vi "UI_Set_Stop_State_(04A).vi"(3 "error in (no error)":errorcluster, 4 "Settings cluster in":T1={"Defaults"={"Default User"=0.0, "VISA Resource Name "=""}, "Recording and saving"={"Researcher name"="", "Name prefix"="", "Data filtering"=0, "Stop at"=0.0, "\"Stop at\" enabled"=FALSE}, "Geometry"={"Cage diameter, mm"=0, "Starting angle MIDFIELD"=0, "Starting angle BORDER"=0, "Radius, mm CENTER"=0, "Radius, mm MIDFIELD"=0, "N segments MIDFIELD"=0, "N segments BORDER"=0, "R-gap, mm"=0.0, "Bridge swap"=FALSE, "Bridge H. offset"=0.0, "Bridge V. offset"=0.0, "Twisted neck"=FALSE, "Alt. magn. orientation"=FALSE}, "IO parameters"={"IO general config."=0, "IO 1 configuration"=0, "IO 2 configuration"=0, "IO 3 configuration"=0, "IO 4 configuration"=0, "Activate ext. RS-232"=0, "IO inversion config."=0, "Sync capability"=1}, "Stimulus presets array"=[{"Event type"=0, "Dur., s"=0.0, "Stim., s"=0.0, "TTL out N"=1, "Set/Clear"=FALSE, "Stim. has been set"=FALSE}, {"Event type"=0, "Dur., s"=0.0, "Stim., s"=0.0, "TTL out N"=1, "Set/Clear"=FALSE, "Stim. has been set"=FALSE}, {"Event type"=0, "Dur., s"=0.0, "Stim., s"=0.0, "TTL out N"=1, "Set/Clear"=FALSE, "Stim. has been set"=FALSE}, {"Event type"=0, "Dur., s"=0.0, "Stim., s"=0.0, "TTL out N"=1, "Set/Clear"=FALSE, "Stim. has been set"=FALSE}, {"Event type"=0, "Dur., s"=0.0, "Stim., s"=0.0, "TTL out N"=1, "Set/Clear"=FALSE, "Stim. has been set"=FALSE}, {"Event type"=0, "Dur., s"=0.0, "Stim., s"=0.0, "TTL out N"=1, "Set/Clear"=FALSE, "Stim. has been set"=FALSE}, {"Event type"=0, "Dur., s"=0.0, "Stim., s"=0.0, "TTL out N"=1, "Set/Clear"=FALSE, "Stim. has been set"=FALSE}, {"Event type"=0, "Dur., s"=0.0, "Stim., s"=0.0, "TTL out N"=1, "Set/Clear"=FALSE, "Stim. has been set"=FALSE}, {"Event type"=0, "Dur., s"=0.0, "Stim., s"=0.0, "TTL out N"=1, "Set/Clear"=FALSE, "Stim. has been set"=FALSE}, {"Event type"=0, "Dur., s"=0.0, "Stim., s"=0.0, "TTL out N"=1, "Set/Clear"=FALSE, "Stim. has been set"=FALSE}, {"Event type"=0, "Dur., s"=0.0, "Stim., s"=0.0, "TTL out N"=1, "Set/Clear"=FALSE, "Stim. has been set"=FALSE}, {"Event type"=0, "Dur., s"=0.0, "Stim., s"=0.0, "TTL out N"=1, "Set/Clear"=FALSE, "Stim. has been set"=FALSE}, {"Event type"=0, "Dur., s"=0.0, "Stim., s"=0.0, "TTL out N"=1, "Set/Clear"=FALSE, "Stim. has been set"=FALSE}, {"Event type"=0, "Dur., s"=0.0, "Stim., s"=0.0, "TTL out N"=1, "Set/Clear"=FALSE, "Stim. has been set"=FALSE}], "Settings loaded OK"=FALSE} {"Stimulus presets array"."Event type" items=["Stay for N seconds"]; "Stimulus presets array"."TTL out N" items=["1"=1, "2"=2, "1+2"=3]; "Geometry"."Cage diameter, mm" scale=0.0..340.0}, 5 "All references in":T7) -> (0 "error out":errorcluster, 1 "Settings cluster out":T1={"Defaults"={"Default User"=0.0, "VISA Resource Name "=""}, "Recording and saving"={"Researcher name"="", "Name prefix"="", "Data filtering"=0, "Stop at"=0.0, "\"Stop at\" enabled"=FALSE}, "Geometry"={"Cage diameter, mm"=0, "Starting angle MIDFIELD"=0, "Starting angle BORDER"=0, "Radius, mm CENTER"=0, "Radius, mm MIDFIELD"=0, "N segments MIDFIELD"=0, "N segments BORDER"=0, "R-gap, mm"=0.0, "Bridge swap"=FALSE, "Bridge H. offset"=0.0, "Bridge V. offset"=0.0, "Twisted neck"=FALSE, "Alt. magn. orientation"=FALSE}, "IO parameters"={"IO general config."=0, "IO 1 configuration"=0, "IO 2 configuration"=0, "IO 3 configuration"=0, "IO 4 configuration"=0, "Activate ext. RS-232"=0, "IO inversion config."=0, "Sync capability"=1}, "Stimulus presets array"=[{"Event type"=0, "Dur., s"=0.0, "Stim., s"=0.0, "TTL out N"=1, "Set/Clear"=FALSE, "Stim. has been set"=FALSE}, {"Event type"=0, "Dur., s"=0.0, "Stim., s"=0.0, "TTL out N"=1, "Set/Clear"=FALSE, "Stim. has been set"=FALSE}, {"Event type"=0, "Dur., s"=0.0, "Stim., s"=0.0, "TTL out N"=1, "Set/Clear"=FALSE, "Stim. has been set"=FALSE}, {"Event type"=0, "Dur., s"=0.0, "Stim., s"=0.0, "TTL out N"=1, "Set/Clear"=FALSE, "Stim. has been set"=FALSE}, {"Event type"=0, "Dur., s"=0.0, "Stim., s"=0.0, "TTL out N"=1, "Set/Clear"=FALSE, "Stim. has been set"=FALSE}, {"Event type"=0, "Dur., s"=0.0, "Stim., s"=0.0, "TTL out N"=1, "Set/Clear"=FALSE, "Stim. has been set"=FALSE}, {"Event type"=0, "Dur., s"=0.0, "Stim., s"=0.0, "TTL out N"=1, "Set/Clear"=FALSE, "Stim. has been set"=FALSE}, {"Event type"=0, "Dur., s"=0.0, "Stim., s"=0.0, "TTL out N"=1, "Set/Clear"=FALSE, "Stim. has been set"=FALSE}, {"Event type"=0, "Dur., s"=0.0, "Stim., s"=0.0, "TTL out N"=1, "Set/Clear"=FALSE, "Stim. has been set"=FALSE}, {"Event type"=0, "Dur., s"=0.0, "Stim., s"=0.0, "TTL out N"=1, "Set/Clear"=FALSE, "Stim. has been set"=FALSE}, {"Event type"=0, "Dur., s"=0.0, "Stim., s"=0.0, "TTL out N"=1, "Set/Clear"=FALSE, "Stim. has been set"=FALSE}, {"Event type"=0, "Dur., s"=0.0, "Stim., s"=0.0, "TTL out N"=1, "Set/Clear"=FALSE, "Stim. has been set"=FALSE}, {"Event type"=0, "Dur., s"=0.0, "Stim., s"=0.0, "TTL out N"=1, "Set/Clear"=FALSE, "Stim. has been set"=FALSE}, {"Event type"=0, "Dur., s"=0.0, "Stim., s"=0.0, "TTL out N"=1, "Set/Clear"=FALSE, "Stim. has been set"=FALSE}], "Settings loaded OK"=FALSE} {"Stimulus presets array"."Event type" items=["Stay for N seconds"]; "Stimulus presets array"."TTL out N" items=["1"=1, "2"=2, "1+2"=3]; "Geometry"."Cage diameter, mm" scale=0.0..340.0}, 2 "All references out":T7)   [LabVIEW 2018]
uses:
  Controls/CTL_All_References.ctl
  Controls/CTL_Controls_References.ctl
  Controls/CTL_Indicators_References.ctl
  Controls/CTL_Panes_and_VIs_References.ctl
  Controls/CTL_Histogram_Properties.ctl
  <vilib>/Utility/miscctls.llb/LVRangeTypeDef.ctl
  Controls/CTL_Settings_cluster.ctl
  Controls/CTL_Segmented_plot_parameters.ctl
  Controls/CTL_IO_params_cluster.ctl
  Controls/CTL_Single_stimulus_setting.ctl
  <vilib>/Utility/error.llb/Error Cluster From Error Code.vi
  <vilib>/ErrorRing/Error Ring.xnode
panel:
  in  "Histogram initialization cluster":T5={"X Scale.Range"={"Minimum"=0.0, "Maximum"=13.0, "Increment"=1.0, "Minor Increment"=1.0, "Start"=0.0}, "Caption.Text"="Zone preference (normalized)", "X Scale.Offset and Multiplier:Multiplier"=1.0, "X Scale.Offset and Multiplier:Offset"=0.0, "X Scale.Scale Fit"=2, "X Scale.Display Format:Precision"=0, "Y Scale.Mapping Mode"=0, "Zones preference empty initialized array"=[0, 0, 0, 0, 0, 0, 0, 0, 0, 0, 0, 0, 0, 0], "Plot.Fill/Point Color"=15790320}
  out "Panes references":T10
  out "Controls references params":string[][](array[string])
  out "Indicators references params":string[][](array[string])
  out "Indicators references":T9
  out "Controls references":T8
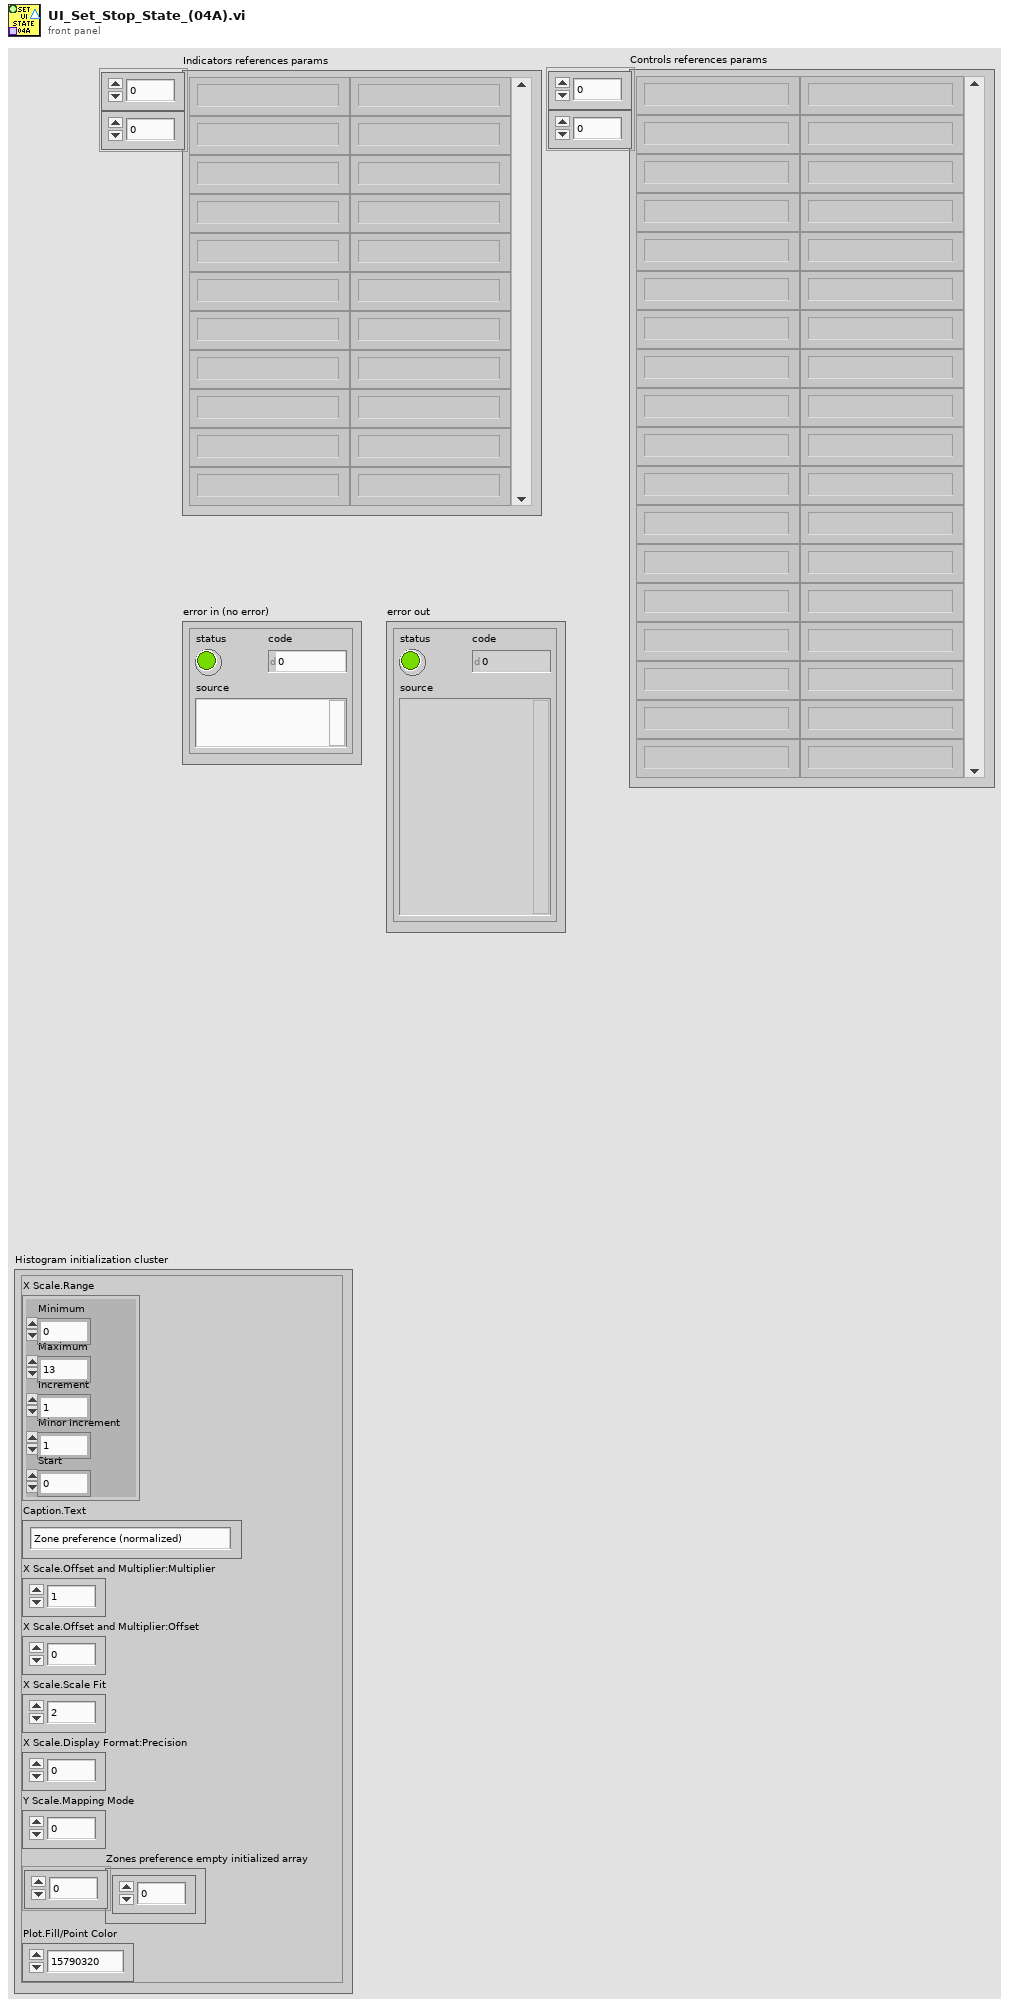
[diagram p1: front panel]
types:
  T1 = typedef "CTL_Settings_cluster.ctl" = cluster{"Defaults":cluster{"Default User":dbl, "VISA Resource Name ":string}, "Recording and saving":cluster{"Researcher name":string, "Name prefix":string, "Data filtering":u16, "Stop at":dbl, "\"Stop at\" enabled":bool}, "Geometry":T2, "IO parameters":T3, "Stimulus presets array":T4[], "Settings loaded OK":bool}
  T2 = typedef "CTL_Segmented_plot_parameters.ctl" = cluster{"Cage diameter, mm":u16, "Starting angle MIDFIELD":i16, "Starting angle BORDER":i16, "Radius, mm CENTER":u16, "Radius, mm MIDFIELD":u16, "N segments MIDFIELD":u8, "N segments BORDER":u8, "R-gap, mm":sgl, "Bridge swap":bool, "Bridge H. offset":sgl, "Bridge V. offset":sgl, "Twisted neck":bool, "Alt. magn. orientation":bool}
  T3 = typedef "CTL_IO_params_cluster.ctl" = cluster{"IO general config.":u16, "IO 1 configuration":u16, "IO 2 configuration":u16, "IO 3 configuration":u16, "IO 4 configuration":u16, "Activate ext. RS-232":u16, "IO inversion config.":u16, "Sync capability":u8}
  T4 = typedef "CTL_Single_stimulus_setting.ctl" = cluster{"Event type":u16, "Dur., s":sgl, "Stim., s":sgl, "TTL out N":u16, "Set/Clear":bool, "Stim. has been set":bool}
  T5 = typedef "CTL_Histogram_Properties.ctl" = cluster{"X Scale.Range":T6, "Caption.Text":string, "X Scale.Offset and Multiplier:Multiplier":dbl, "X Scale.Offset and Multiplier:Offset":dbl, "X Scale.Scale Fit":u8, "X Scale.Display Format:Precision":u8, "Y Scale.Mapping Mode":u8, "Zones preference empty initialized array":i32[], "Plot.Fill/Point Color":u32}
  T6 = typedef "LVRangeTypeDef.ctl" = cluster{"Minimum":dbl, "Maximum":dbl, "Increment":dbl, "Minor Increment":dbl, "Start":dbl}
  T7 = typedef "CTL_All_References.ctl" = cluster{"Controls references":T8, "Indicators references":T9, "Panes references":T10}
  T8 = typedef "CTL_Controls_References.ctl" = cluster{"Check HW connection":refnum<vi>, "Start Tracking button":refnum<vi>, "Reset zones":refnum<vi>, "Reset stimuli":refnum<vi>, "Record/Stop":refnum<vi>, "Reset barplot":refnum<vi>, "Multiplyer of chart RX":refnum<vi>, "Show zones":refnum<vi>, "Show magnets":refnum<vi>, "Show heatmap":refnum<vi>, "Show full track":refnum<vi>, "Open File":refnum<vi>, "Play/Pause":refnum<vi>, "Trace, s":refnum<vi>, "Playback speed":refnum<vi>, "Timeline":refnum<vi>, "By Zone stim. setup":refnum<vi>, "Set, Rec and Analyse Tab":refnum<vi>, "Cage radial segmentation":refnum<vi>, "Set IO config":refnum<vi>}
  T9 = typedef "CTL_Indicators_References.ctl" = cluster{"HW info":refnum<vi>, "Port":refnum<vi>, "Ready":refnum<vi>, "IO status indicator":refnum<vi>, "Current Time":refnum<vi>, "Record timestamp":refnum<vi>, "Mouse speed":refnum<vi>, "Mouse speed, mm/s":refnum<vi>, "Running, perc. of time":refnum<vi>, "Histograms":refnum<vi>, "Cage size":refnum<vi>}
  T10 = typedef "CTL_Panes_and_VIs_References.ctl" = cluster{"Pane":refnum<vi>, "This VI":refnum<vi>}
  T11 = enum8{"Enabled", "Disabled", "Disabled and Grayed Out"}
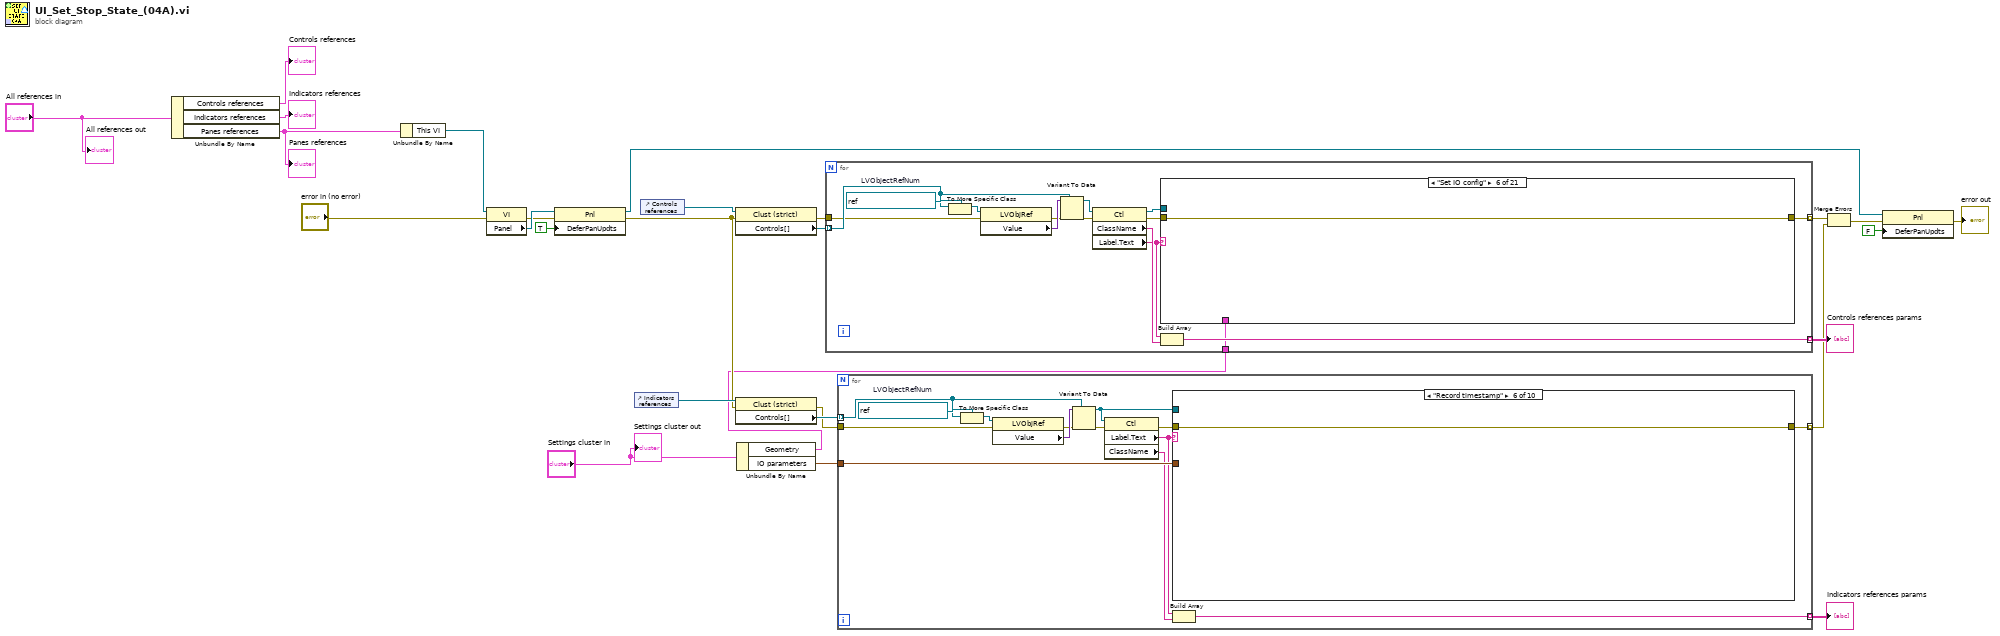
[diagram p0: block diagram]
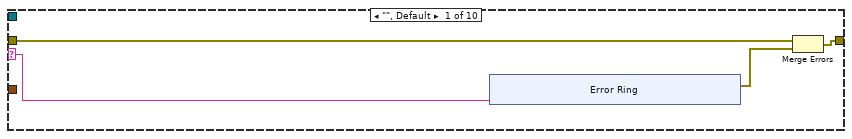
[diagram p2: hidden frame]
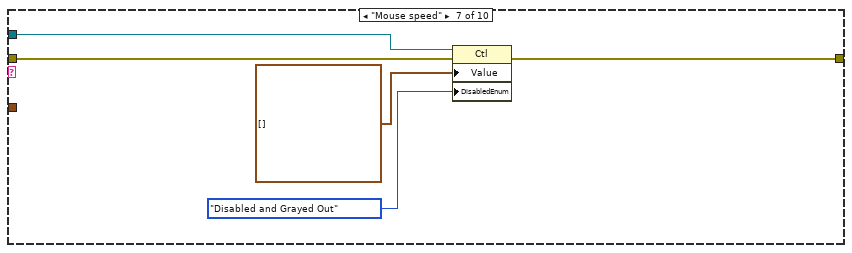
[diagram p7: hidden frame]
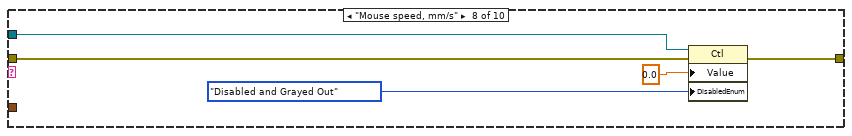
[diagram p8: hidden frame]
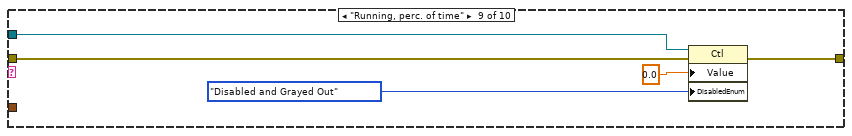
[diagram p9: hidden frame]
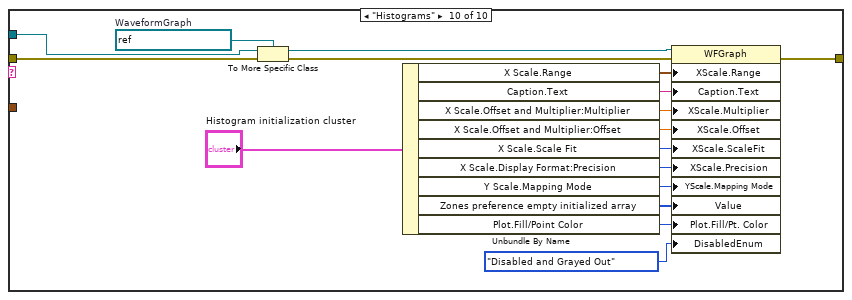
[diagram p10: hidden frame]
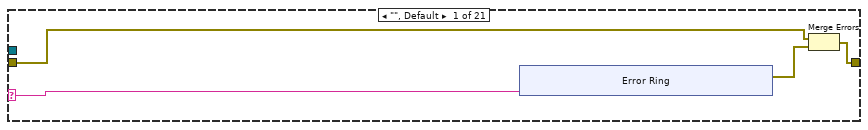
[diagram p11: hidden frame]
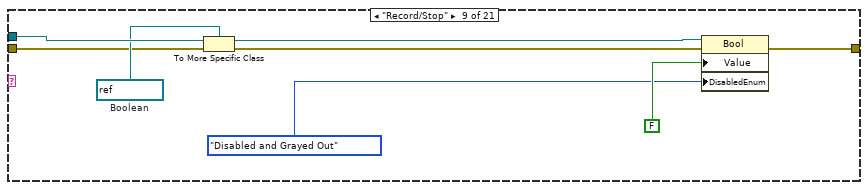
[diagram p18: hidden frame]
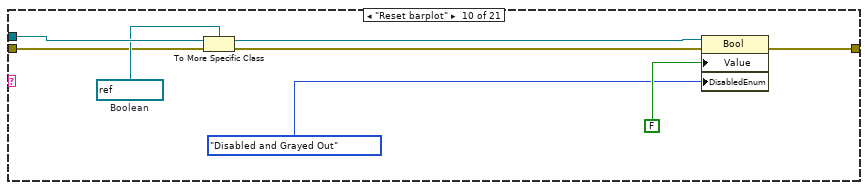
[diagram p19: hidden frame]
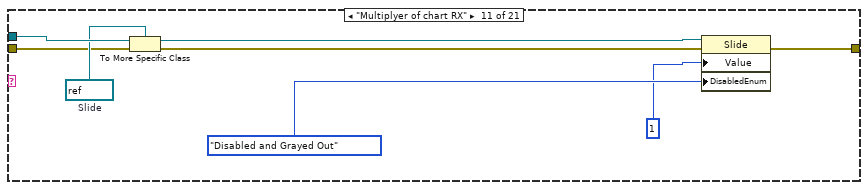
[diagram p20: hidden frame]
diagram:
  n1 = Unbundle By Name("All references in") -> ("Controls references"=→"Controls references":T8, "Indicators references"=→"Indicators references":T9, "Panes references"=w18:T10)
  "Panes references" <- w18
  n2 = Unbundle By Name(w18) -> ("This VI"=w15:refnum<vi>)
  n3 = property class="VI"(reference=w15, error in="error in (no error)") -> (error out=w7:errorcluster, "Panel"=w17:refnum<vi>)  [unwired: 1 out]
  n4 = property class="Pnl"(reference=w17, error in=w7, "DeferPanUpdts"=TRUE ("Defer Panel Updates")) -> (reference out=w8:refnum<vi>, error out=w14:errorcluster)
  n5 = control-ref of="Indicators references"() -> (w21:refnum<vi>)
  n6 = control-ref of="Controls references"() -> (w23:refnum<vi>)
  n7 = property class="Clust (strict)"(reference=w23, error in=w14) -> (error out=w13:errorcluster, "Controls[]"=w24:refnum<vi>[])  [unwired: 1 out]
  n8 = property class="Clust (strict)"(reference=w21, error in=w14) -> (error out=w12:errorcluster, "Controls[]"=w22:refnum<vi>[])  [unwired: 1 out]
  n9 = Unbundle By Name("Settings cluster in") -> ("Geometry"=w1:T2, "IO parameters"=w3:T3)
  n10 = for {
    tunnel: w24 -> [w39] mode=indexing
    tunnel: [w36] -> w19 mode=indexing
    tunnel: w13 -> [w35]
    tunnel: [w31] -> w5 mode=indexing
    tunnel: w1 -> [w28]
    w41 = refnum<vi> refnum  # LVObjectRefNum
    n11 = To More Specific Class(target class=w41, reference=w39) -> (specific class reference=w42:refnum<vi>)  [unwired: 1 in, 1 out]
    n12 = property class="LVObjRef"(reference=w42, error in=w35) -> (error out=w34:errorcluster, "Value"=w40:variant)  [unwired: 1 out]
    n13 = Variant To Data(error in=w34, type=w39, Variant=w40) -> (data=w38:refnum<vi>, error out=w33:errorcluster)
    n14 = property class="Ctl"(reference=w38, error in=w33) -> (reference out=w29:refnum<vi>, error out=w30:errorcluster, "ClassName"=w37:string, "Label.Text"=w32:string)
    n15 = case shown="\"Set IO config\"" w32 {
      selector: w32 -> [w43 _ _ _ _ _ _ _ _ _ _ _ _ _ _ _ _ _ _ _ _]
      tunnel: [w45 w54 w55 w56 w57 w58 w59 w60 w63 w71 w79 w85 w86 w89 w97 w103 w104 w107 w115 w123 w129] -> w31
      tunnel: w30 -> [w46 w54 w55 w56 w57 w58 w59 w60 w65 w73 w81 w85 w86 w91 w99 w103 w104 w109 w117 w125 w129]
      tunnel: w29 -> [_ _ _ _ _ _ _ _ w68 w76 w84 _ _ w94 w102 _ _ w112 w120 w128 _]
      tunnel: w28 -> [_ _ _ _ _ _ _ _ _ _ _ _ _ _ _ _ _ _ _ _ _]
      frame "", Default {
        n16 = xnode "Error Ring"("parameter 0"=w43) -> ("error out"=w44:errorcluster)
        n17 = Merge Errors(w46, w44) -> (w45:errorcluster)
      }
      frame "Cage radial segmentation" {
      }
      frame "Set/Rec and Analyse Tab" {
      }
      frame "Check HW connection" {
      }
      frame "Save settings" {
      }
      frame "Set IO config" {
      }
      frame "Reset zones" {
      }
      frame "Reset stimuli" {
      }
      frame "Record/Stop" {
        w67 = refnum<vi> refnum  # Boolean
        n18 = To More Specific Class(target class=w67, reference=w68, error in=w65) -> (specific class reference=w66:refnum<vi>, error out=w64:errorcluster)
        n19 = property class="Bool"(reference=w66, error in=w64, "Value"=FALSE, "DisabledEnum"=T11."Disabled and Grayed Out" ("Disabled")) -> (error out=w63:errorcluster)  [unwired: 1 out]
      }
      frame "Reset barplot" {
        w75 = refnum<vi> refnum  # Boolean
        n20 = To More Specific Class(target class=w75, reference=w76, error in=w73) -> (specific class reference=w74:refnum<vi>, error out=w72:errorcluster)
        n21 = property class="Bool"(reference=w74, error in=w72, "Value"=FALSE, "DisabledEnum"=T11."Disabled and Grayed Out" ("Disabled")) -> (error out=w71:errorcluster)  [unwired: 1 out]
      }
      frame "Multiplyer of chart RX" {
        w83 = refnum<vi> refnum  # Slide
        n22 = To More Specific Class(target class=w83, reference=w84, error in=w81) -> (specific class reference=w82:refnum<vi>, error out=w80:errorcluster)
        n23 = property class="Slide"(reference=w82, error in=w80, "Value"=u8 1, "DisabledEnum"=T11."Disabled and Grayed Out" ("Disabled")) -> (error out=w79:errorcluster)  [unwired: 1 out]
      }
      frame "Show zones" {
      }
      frame "Show magnets" {
      }
      frame "Show heatmap" {
        w93 = refnum<vi> refnum  # Boolean
        n24 = To More Specific Class(target class=w93, reference=w94, error in=w91) -> (specific class reference=w92:refnum<vi>, error out=w90:errorcluster)
        n25 = property class="Bool"(reference=w92, error in=w90, "Value"=FALSE, "DisabledEnum"=T11."Disabled and Grayed Out" ("Disabled")) -> (error out=w89:errorcluster)  [unwired: 1 out]
      }
      frame "Show full track" {
        w101 = refnum<vi> refnum  # Boolean
        n26 = To More Specific Class(target class=w101, reference=w102, error in=w99) -> (specific class reference=w100:refnum<vi>, error out=w98:errorcluster)
        n27 = property class="Bool"(reference=w100, error in=w98, "Value"=FALSE, "DisabledEnum"=T11."Disabled and Grayed Out" ("Disabled")) -> (error out=w97:errorcluster)  [unwired: 1 out]
      }
      frame "Open File" {
      }
      frame "Play/Pause" {
      }
      frame "Trace, s" {
        w111 = refnum<vi> refnum  # Slide
        n28 = To More Specific Class(target class=w111, reference=w112, error in=w109) -> (specific class reference=w110:refnum<vi>, error out=w108:errorcluster)
        n29 = property class="Slide"(reference=w110, error in=w108, "Value"=u8 5, "DisabledEnum"=T11."Disabled and Grayed Out" ("Disabled")) -> (error out=w107:errorcluster)  [unwired: 1 out]
      }
      frame "Playback speed" {
        w119 = refnum<vi> refnum  # Ring
        n30 = To More Specific Class(target class=w119, reference=w120, error in=w117) -> (specific class reference=w118:refnum<vi>, error out=w116:errorcluster)
        n31 = property class="Ring"(reference=w118, error in=w116, "Value"=u8 3, "DisabledEnum"=T11."Disabled and Grayed Out" ("Disabled")) -> (error out=w115:errorcluster)  [unwired: 1 out]
      }
      frame "Timeline" {
        w127 = refnum<vi> refnum  # Slide
        n32 = To More Specific Class(target class=w127, reference=w128, error in=w125) -> (specific class reference=w126:refnum<vi>, error out=w124:errorcluster)
        n33 = property class="Slide"(reference=w126, error in=w124, "Value"=u8 5, "DisabledEnum"=T11."Disabled and Grayed Out" ("Disabled")) -> (error out=w123:errorcluster)  [unwired: 1 out]
      }
      frame "By Zone stim. setup" {
      }
    }
    n34 = Build Array(w32, w37) -> (w36:string[])
  }
  "Controls references params" <- w19
  n35 = for {
    tunnel: w22 -> [w140] mode=indexing
    tunnel: [w130] -> w20 mode=indexing
    tunnel: w12 -> [w138]
    tunnel: [w134] -> w11 mode=indexing
    tunnel: w3 -> [w133]
    w142 = refnum<vi> refnum  # LVObjectRefNum
    n36 = To More Specific Class(target class=w142, reference=w140) -> (specific class reference=w143:refnum<vi>)  [unwired: 1 in, 1 out]
    n37 = property class="LVObjRef"(reference=w143, error in=w138) -> (error out=w137:errorcluster, "Value"=w141:variant)  [unwired: 1 out]
    n38 = Variant To Data(error in=w137, type=w140, Variant=w141) -> (data=w139:refnum<vi>, error out=w136:errorcluster)
    n39 = property class="Ctl"(reference=w139, error in=w136) -> (error out=w135:errorcluster, "Label.Text"=w132:string, "ClassName"=w131:string)  [unwired: 1 out]
    n40 = case shown="\"Record timestamp\"" w132 {
      selector: w132 -> [w144 _ _ _ _ _ _ _ _ _]
      tunnel: w139 -> [_ _ _ _ _ _ w164 w169 w174 w191]
      tunnel: w135 -> [w147 w155 w156 w157 w158 w159 w163 w168 w173 w177]
      tunnel: [w146 w155 w156 w157 w158 w159 w162 w167 w172 w190] -> w134
      tunnel: w133 -> [_ _ _ _ _ _ _ _ _ _]
      frame "", Default {
        n41 = xnode "Error Ring"("parameter 0"=w144) -> ("error out"=w145:errorcluster)
        n42 = Merge Errors(w147, w145) -> (w146:errorcluster)
      }
      frame "Cage size", "HW info", "Port" {
      }
      frame "Ready" {
      }
      frame "IO status indicator" {
      }
      frame "Current Time" {
      }
      frame "Record timestamp" {
      }
      frame "Mouse speed" {
        n43 = property class="Ctl"(reference=w164, error in=w163, "Value"=waveform(dbl)[] [] ("History Data"), "DisabledEnum"=T11."Disabled and Grayed Out" ("Disabled")) -> (error out=w162:errorcluster)  [unwired: 1 out]
      }
      frame "Mouse speed, mm/s" {
        n44 = property class="Ctl"(reference=w169, error in=w168, "Value"=0.0, "DisabledEnum"=T11."Disabled and Grayed Out" ("Disabled")) -> (error out=w167:errorcluster)  [unwired: 1 out]
      }
      frame "Running, perc. of time" {
        n45 = property class="Ctl"(reference=w174, error in=w173, "Value"=0.0, "DisabledEnum"=T11."Disabled and Grayed Out" ("Disabled")) -> (error out=w172:errorcluster)  [unwired: 1 out]
      }
      frame "Histograms" {
        w188 = refnum<vi> refnum  # WaveformGraph
        n46 = To More Specific Class(target class=w188, reference=w191, error in=w177) -> (specific class reference=w189:refnum<vi>, error out=w176:errorcluster)
        n47 = Unbundle By Name("Histogram initialization cluster") -> ("X Scale.Range"=w186:T6, "Caption.Text"=w185:string, "X Scale.Offset and Multiplier:Multiplier"=w184:dbl, "X Scale.Offset and Multiplier:Offset"=w183:dbl, "X Scale.Scale Fit"=w182:u8, "X Scale.Display Format:Precision"=w181:u8, "Y Scale.Mapping Mode"=w180:u8, "Zones preference empty initialized array"=w179:i32[], "Plot.Fill/Point Color"=w178:u32)
        n48 = property class="WFGraph"(reference=w189, error in=w176, "XScale.Range"=w186, "Caption.Text"=w185, "XScale.Multiplier"=w184, "XScale.Offset"=w183, "XScale.ScaleFit"=w182, "XScale.Precision"=w181, "YScale.Mapping Mode"=w180, "Value"=w179, "Plot.Fill/Pt. Color"=w178, "DisabledEnum"=T11."Disabled and Grayed Out" ("Disabled")) -> (error out=w190:errorcluster)  [unwired: 1 out]
      }
    }
    n49 = Build Array(w132, w131) -> (w130:string[])
  }
  "Indicators references params" <- w20
  n50 = Merge Errors(w5, w11) -> (w10:errorcluster)
  n51 = property class="Pnl"(reference=w8, error in=w10, "DeferPanUpdts"=FALSE ("Defer Panel Updates")) -> (error out=→"error out":errorcluster)  [unwired: 1 out]
  "All references out" <- "All references in"
  "Settings cluster out" <- "Settings cluster in"
